vi "RP IV pattern write.vi"(4 "no bram":bool, 8 "Error In":errorcluster, 9 "Waveform parameters":T1={"Start magnitude"=1000.0, "Magnitude increment"=1000.0, "Number of pulses"=8, "Ramp length"=32, "Top  length"=480, "Threshold "=3000, "Processing delay"=240, "Stop after"=1, "Detector window"=480} {"Detector window" format="%dpts"; "Stop after" format="%d sweep(s)"}, 11 "connection ID":refnum<k5>) -> (0 "Error Out":errorcluster, 3 "connection ID out":refnum<k5>, 5 "Waveform Graph":i16[](graph))   [LabVIEW 2019]
uses:
  Waform generation/Waveform parameters.ctl
  RP Command.ctl
  RP Write Command TCP.vi
panel:
  in  "Pattern":enum16{"Sine ramp", "Square"}(ring)
  out "Waveform length":u32=2048
  in  "Config offset":u64=20
  out "Step length":u32=2048
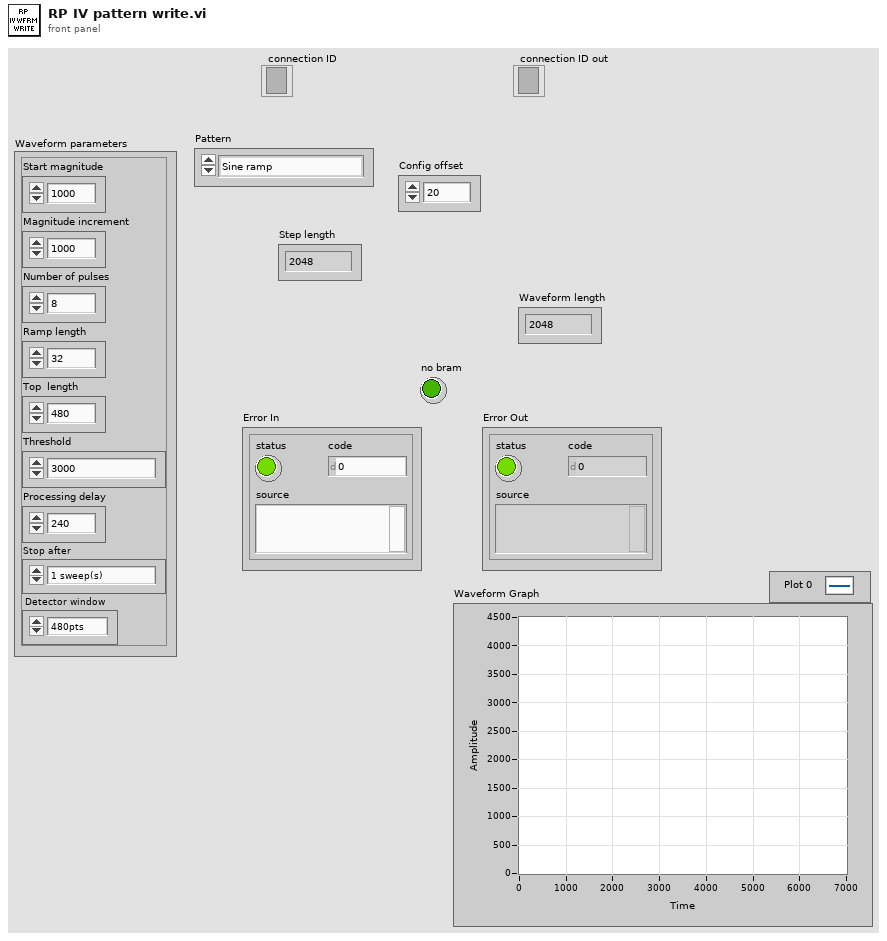
[diagram p1: front panel]
types:
  T1 = typedef "Waveform parameters.ctl" = cluster{"Start magnitude":dbl, "Magnitude increment":dbl, "Number of pulses":i32, "Ramp length":i32, "Top  length":i32, "Threshold ":i32, "Processing delay":u16, "Stop after":u16, "Detector window":i32}
  T2 = typedef "RP Command.ctl" = enum16{"Reset", "Read IDN", "Stop server", "Get status", "Get temperature", "Connect client", "Arm", "Software trigger", "Get whole buffer", "Get chunk", "System call", "Get config", "Set config", "Recieve data", "Recieve Calibartion", "Transmit data"}
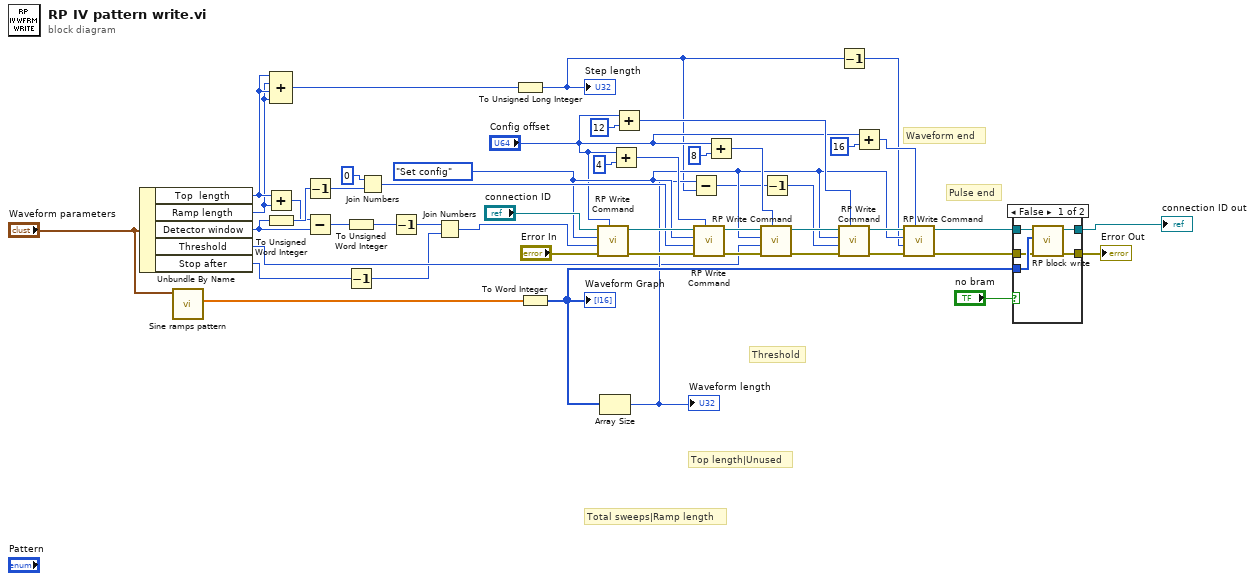
[diagram p0: block diagram]
diagram:
  w30 = RP_Command."Set config" ("Command number")
  # "Pulse end"
  # "Waveform end"
  # "Threshold"
  # "Top length|Unused"
  # "Total sweeps|Ramp length"
  n1 = Unbundle By Name("Waveform parameters") -> ("Top  length"=w5:i32, "Ramp length"=w4:i32, "Detector window"=w1:i32, "Threshold"=w15:i32, "Stop after"=w11:u16)
  n2 = call "Sine ramps pattern.vi"("Waveform parameters 2"="Waveform parameters") -> ("Waveform"=w20:dbl[])  [unwired: 8 in, 1 out]
  n3 = Add(x=w5, y=w4) -> (x+y=w3:i32)
  n4 = To Unsigned Word Integer(number=w1) -> (unsigned 16bit integer=w16:u16)
  n5 = Compound Arithmetic op=ADD(w5, w4, w5, w4) -> (w13:i32)
  n6 = Decrement(x=w16) -> (x-1=w9:u16)
  n7 = Subtract(x=w3, y=w1) -> (x-y=w2:i32)
  n8 = To Unsigned Word Integer(number=w2) -> (unsigned 16bit integer=w17:u16)
  n9 = Decrement(x=w11) -> (x-1=w6:u16)
  n10 = Join Numbers(hi=u16 0, lo=w9) -> ((hi.lo)=w45:u32)
  n11 = Decrement(x=w17) -> (x-1=w10:u16)
  n12 = Join Numbers(hi=w10, lo=w6) -> ((hi.lo)=w48:u32)
  n13 = To Unsigned Long Integer(number=w13) -> (unsigned 32bit integer=w12:u32)
  "Step length" <- w12
  n14 = To Word Integer(number=w20) -> (16bit integer=w19:i16[])
  "Waveform Graph" <- w19
  n15 = call-poly "RP Write Command.vi"("Config offset"="Config offset", "Error In"="Error In", "Command payload"=w48, "Command number"=w30, "connection ID"="connection ID") -> ("Error Out"=w44:errorcluster, "connection ID out"=w47:refnum<k5>)  [unwired: 4 in, 1 out]
  n16 = Array Size(array=w19) -> (size(s)=w18:i32)
  "Waveform length" <- w18
  n17 = Add(x="Config offset", y=u64 4) -> (x+y=w41:u64)
  n18 = Add(x="Config offset", y=u64 12) -> (x+y=w33:u64)
  n19 = Subtract(x=w18, y=w12) -> (x-y=w14:u32)
  n20 = call-poly "RP Write Command.vi"("Config offset"=w41, "Error In"=w44, "Command payload"=w45, "Command number"=w30, "connection ID"=w47) -> ("Error Out"=w39:errorcluster, "connection ID out"=w40:refnum<k5>)  [unwired: 4 in, 1 out]
  n21 = Add(x="Config offset", y=u64 8) -> (x+y=w37:u64)
  n22 = call-poly "RP Write Command.vi"("Config offset"=w37, "Error In"=w39, "Command payload"=w15, "Command number"=w30, "connection ID"=w40) -> ("Error Out"=w36:errorcluster, "connection ID out"=w35:refnum<k5>)  [unwired: 4 in, 1 out]
  n23 = Decrement(x=w14) -> (x-1=w8:u32)
  n24 = Decrement(x=w12) -> (x-1=w7:u32)
  n25 = call-poly "RP Write Command.vi"("Config offset"=w33, "Error In"=w36, "Command payload"=w8, "Command number"=w30, "connection ID"=w35) -> ("Error Out"=w32:errorcluster, "connection ID out"=w31:refnum<k5>)  [unwired: 4 in, 1 out]
  n26 = Add(x="Config offset", y=u64 16) -> (x+y=w27:u64)
  n27 = call-poly "RP Write Command.vi"("Config offset"=w27, "Error In"=w32, "Command payload"=w7, "Command number"=w30, "connection ID"=w31) -> ("Error Out"=w25:errorcluster, "connection ID out"=w26:refnum<k5>)  [unwired: 4 in, 1 out]
  n28 = case shown="False" "no bram" {
    tunnel: w19 -> [w54 _]
    tunnel: w26 -> [w53 w56]
    tunnel: w25 -> [w52 w55]
    tunnel: [w51 w56] -> w24
    tunnel: [w50 w55] -> w23
    frame False {
      n29 = call "RP block write.vi"("Error In"=w52, "Data"=w54, "connection ID"=w53) -> ("Error Out"=w50:errorcluster, "connection ID out"=w51:refnum<k5>)  [unwired: 7 in]
    }
    frame True {
    }
  }
  "connection ID out" <- w24
  "Error Out" <- w23
